vi "Autonomous Independent.vi"() -> ()   [LabVIEW 2020]
doc: "This VI is called when autonomous begins, and will automatically be terminated when autonomous ends. You can carry out timed or sensor driven robot movement independently without needing to return to the caller."
uses:
  <vilib>/Rock Robotics/WPI/ThirdParty/REV Robotics/REVLib/Typedef/Spark MAX Sensor Type.ctl
  <vilib>/Rock Robotics/WPI/Utilities/WPI_GetSetVariantRefNum.vi
  <vilib>/Rock Robotics/Network Tables/NT Read String.vi
  <vilib>/Rock Robotics/Network Tables/NT Write Numeric Array.vi
  <vilib>/Rock Robotics/Network Tables/NT Write Number.vi
  Robot Global Data.vi
  <vilib>/Rock Robotics/WPI/RobotDrive/WPI_RobotDriveArcadeDrive_Standard(NoSaturation).vi
  <vilib>/Rock Robotics/WPI/Solenoid/WPI_SolenoidValue.ctl
  <vilib>/Rock Robotics/WPI/Solenoid/WPI_SolenoidSetEnum.vi
panel:
  out "Real Yaw 2":dbl
  out "Right Drive Encoder 3":dbl format="%#.3f"
  out "Sensor Position 3":dbl
  out "Timestamp 3":u32
  out "Right Drive Encoder 2":dbl format="%#.3f"
  out "Sensor Position 2":dbl
  out "Timestamp 2":u32
  out "Sensor Position":dbl
  out "Timestamp":u32
  in  "error in 2":errorcluster
  out "Real Yaw":dbl
  out "Right Drive Encoder":dbl format="%#.3f"
  in  "error in":errorcluster
  # "Be sure to right-click and choose Data Operations>>Make Current Value default if you want to save the array values with the VI"
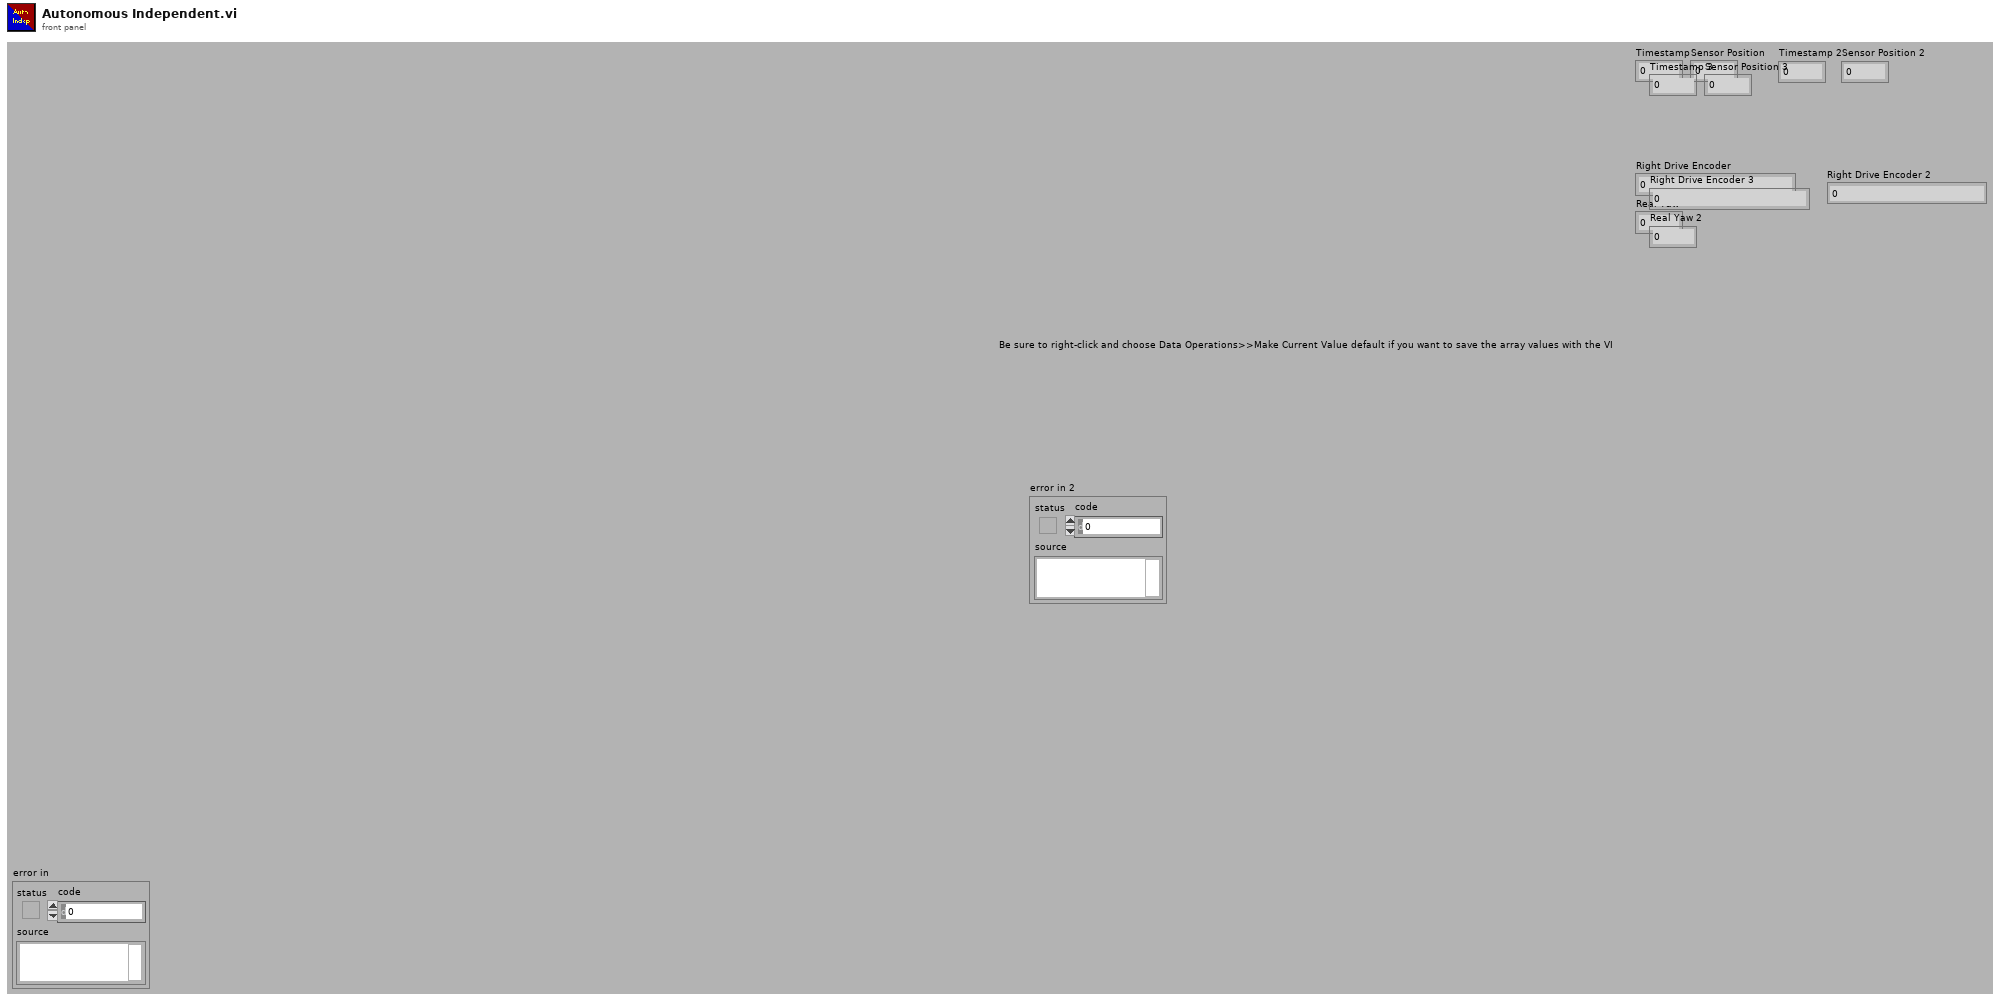
[diagram p1: front panel]
types:
  T1 = typedef "Spark MAX Sensor Type.ctl" = enum16{"No Sensor", "Hall Sensor", "Encoder", "-Not Available-", "Analog", "Alternate Encoder", "Duty Cycle"}
  T2 = typedef "WPI_JoystickDevRef.ctl" = cluster{"Device":T3}
  T3 = typedef "WPI_JoystickDeviceEnum.ctl" = enum16{"USB 0", "USB 1", "USB 2", "USB 3", "USB 4", "USB 5"}
  T4 = typedef "WPI_RobotDriveDevRef.ctl" = cluster{"DevStatus":errorcluster, "Motors[]":T5[], "Square Inputs":bool, "Max Output":dbl}
  T5 = typedef "WPI_MotorControlDeviceRef.ctl" = cluster{"DeviceStatus":errorcluster, "Type":T6, "PWM":cluster{"PWM Channel":T7, "DeadBand":T8}, "CAN":cluster{"Device Number":u8, "SetOutput VI Ref":variant, "GetOutput VI Ref":variant, "Enable VI Ref":variant, "Disable VI Ref":variant, "Data":variant}, "Invert":bool, "DIO PWM":cluster{"PWM \"Enable\" Channel":T7, "DIOChannel":T9, "PWM Rate":dbl}}
  T6 = typedef "WPI_MotorControlType.ctl" = enum16{"PWM", "CAN", "DIO PWM"}
  T7 = typedef "FPGA_DIOPWMChannel.ctl" = enum8{"PWM 0", "PWM 1", "PWM 2", "PWM 3", "PWM 4", "PWM 5", "PWM 6", "PWM 7", "PWM 8", "PWM 9", "PWM MXP 0", "PWM MXP 1", "PWM MXP 2", "PWM MXP 3", "PWM MXP 4", "PWM MXP 5", "PWM MXP 6", "PWM MXP 7", "PWM MXP 8", "PWM MXP 9", "Invalid"}
  T8 = typedef "WPI_PWMDeadband.ctl" = cluster{"Name":string, "maxPositivePwm":i32, "minPositivePwm":i32, "centerPwm":i32, "maxNegativePwm":i32, "minNegativePwm":i32, "angularRange":u16}
  T9 = typedef "FPGA_DIOChannel.ctl" = enum8{"DIO 0", "DIO 1", "DIO 2", "DIO 3", "DIO 4", "DIO 5", "DIO 6", "DIO 7", "DIO 8", "DIO 9", "DIO MXP 0", "DIO MXP 1", "DIO MXP 2", "DIO MXP 3", "DIO MXP 4", "DIO MXP 5", "DIO MXP 6", "DIO MXP 7", "DIO MXP 8", "DIO MXP 9", "DIO MXP 10", "DIO MXP 11", "DIO MXP 12", "DIO MXP 13", "DIO MXP 14", "DIO MXP 15", "SPI Port CS1", "SPI Port CS2", "SPI Port CS3", "SPI Port MISO", "SPI Port MOSI", "Invalid"}
  T10 = cluster{"Motors[][0]":T5, "Motors[][1]":T5, "Motors[][2]":T5, "Motors[][3]":T5, "Motors[][4]":T5, "Motors[][5]":T5, "Motors[][6]":T5, "Motors[][7]":T5, "Motors[][8]":T5}
  T11 = typedef "WPI_SolenoidValue.ctl" = enum16{"Off", "On", "Forward", "Reverse"}
  T12 = typedef "WPI_SolenoidDevRef.ctl" = cluster{"DevStatus":errorcluster, "Pneumatics Control Module":u8, "Forward Solenoid Channel":T13, "Reverse Solenoid Channel":T13}
  T13 = typedef "WPI_SolenoidChannel.ctl" = enum8{"Solenoid 0", "Solenoid 1", "Solenoid 2", "Solenoid 3", "Solenoid 4", "Solenoid 5", "Solenoid 6", "Solenoid 7", "Solenoid 8", "Solenoid 9", "Solenoid 10", "Solenoid 11", "Solenoid 12", "Solenoid 13", "Solenoid 14", "Solenoid 15", "Invalid"}
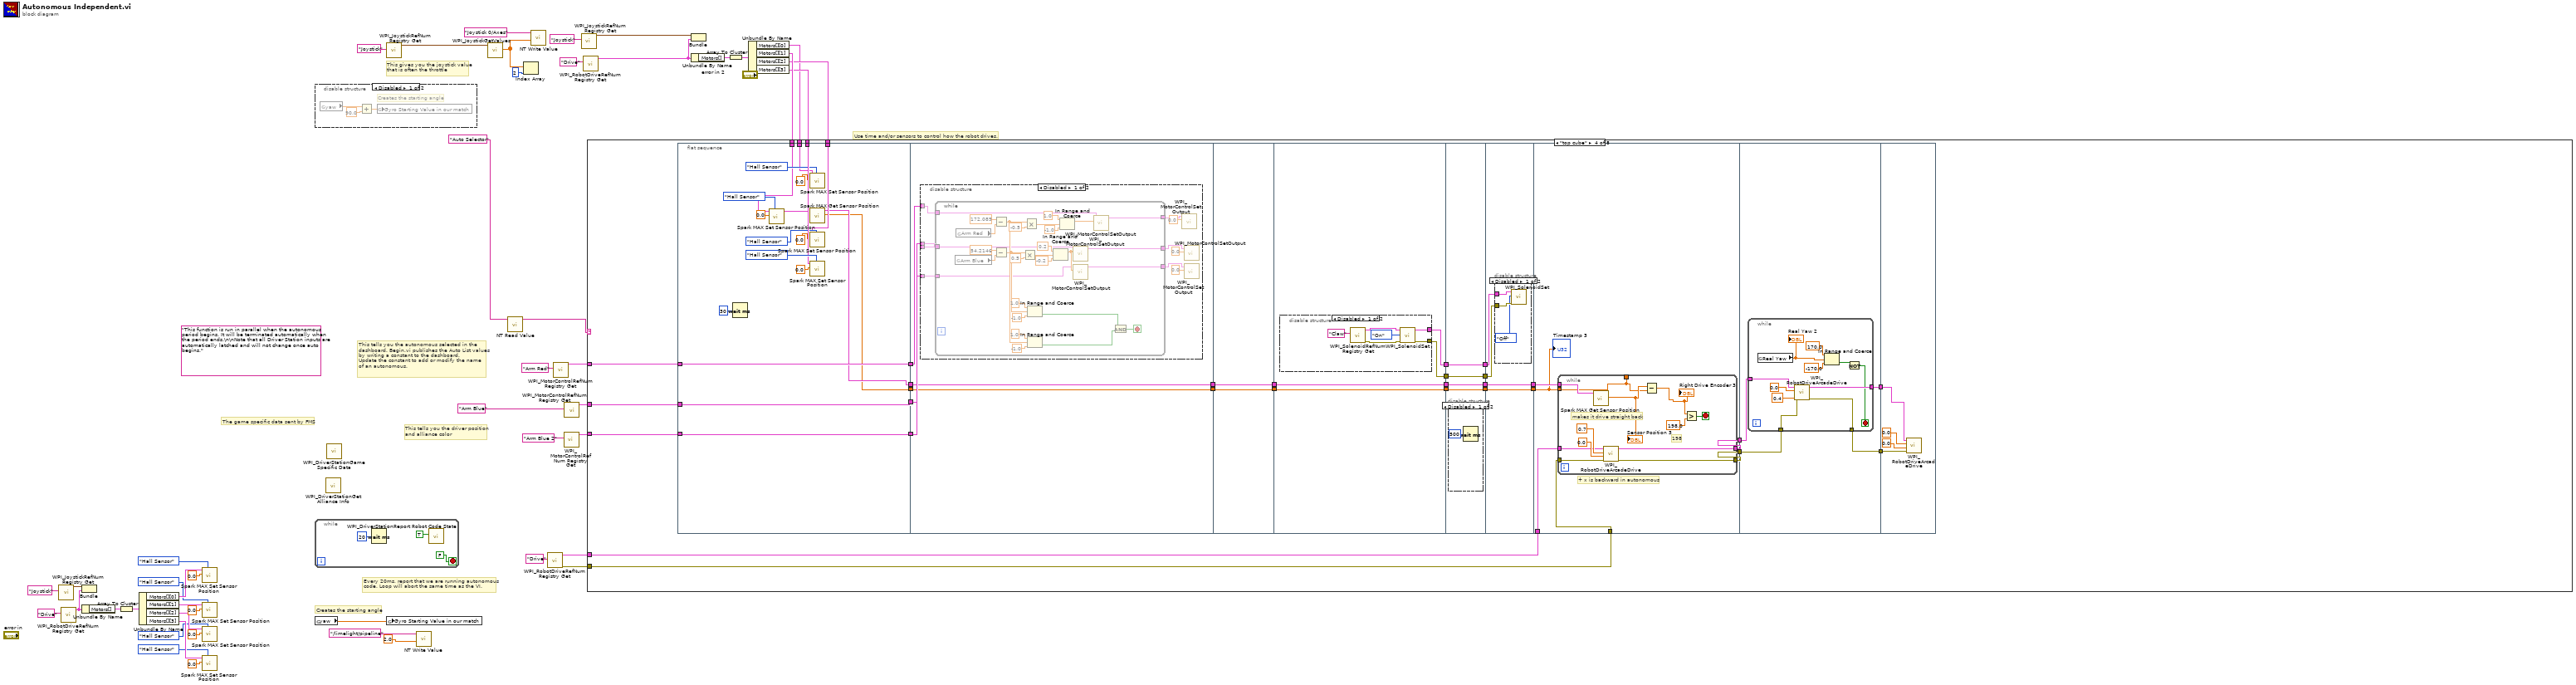
[diagram p0: block diagram]
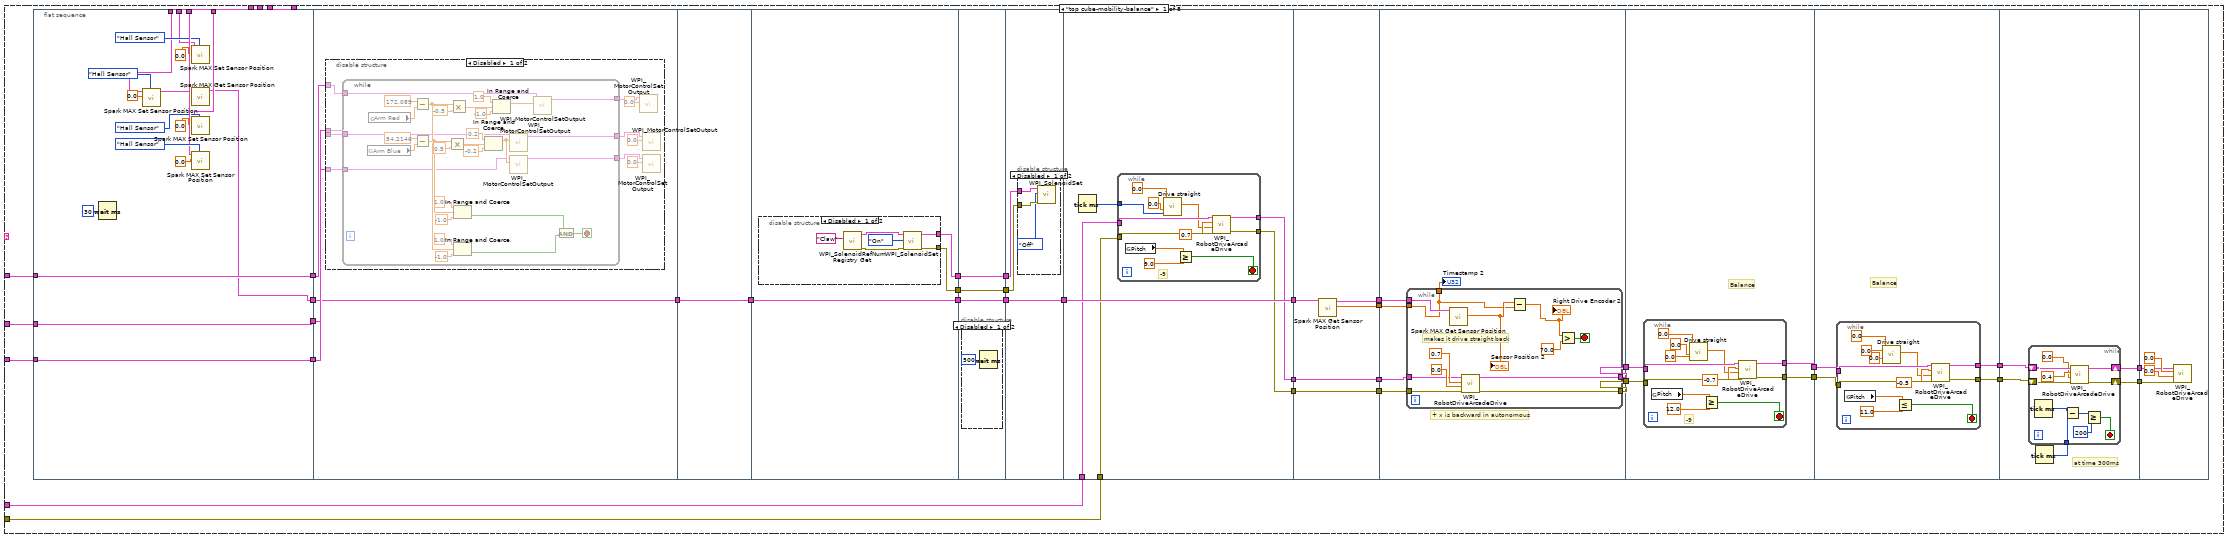
[diagram p3: hidden frame]
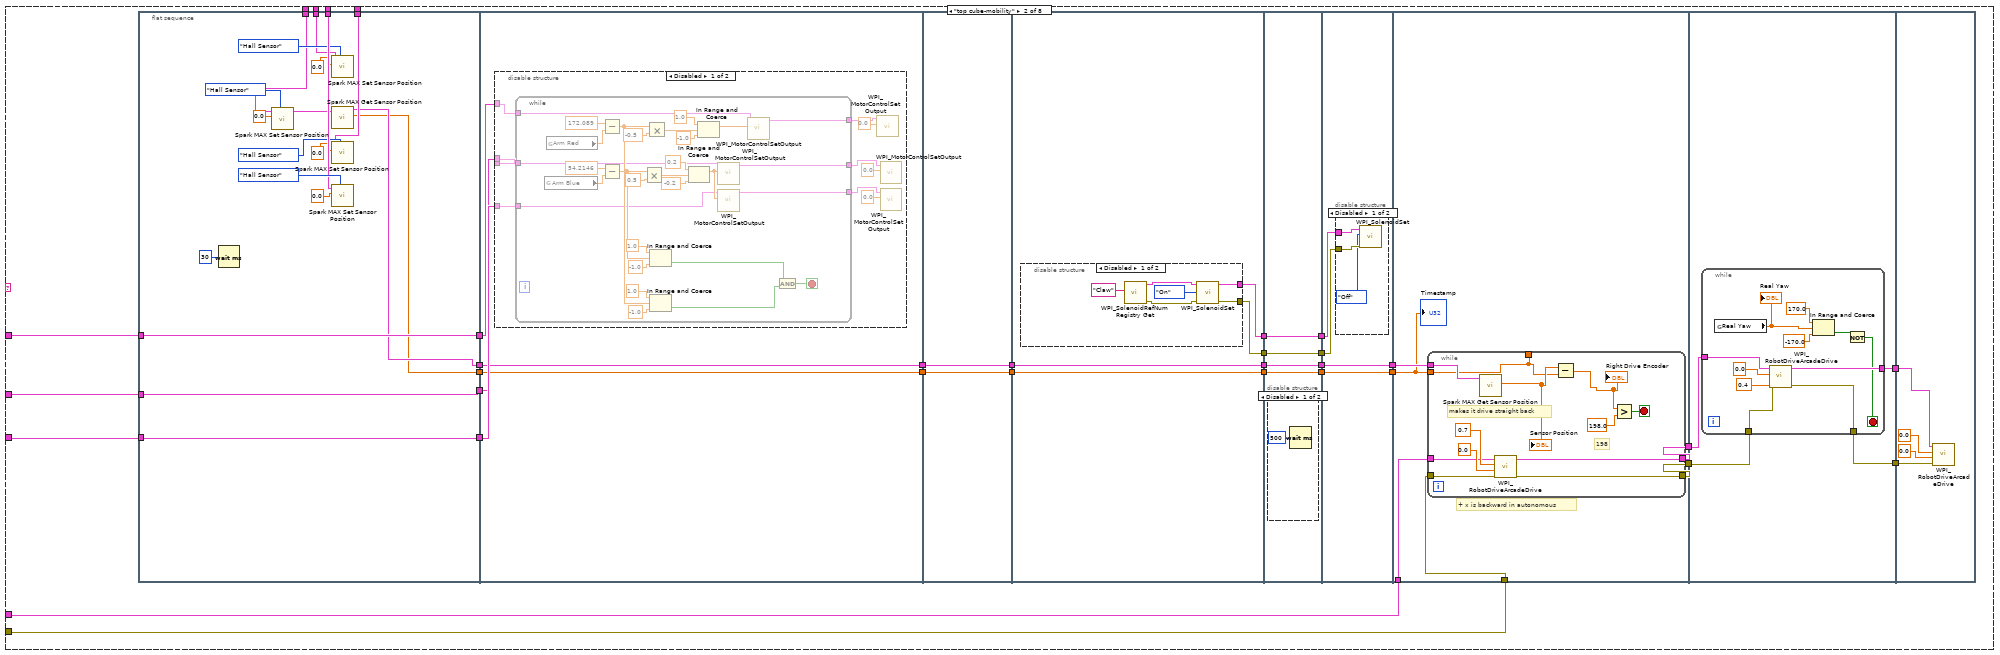
[diagram p8: hidden frame]
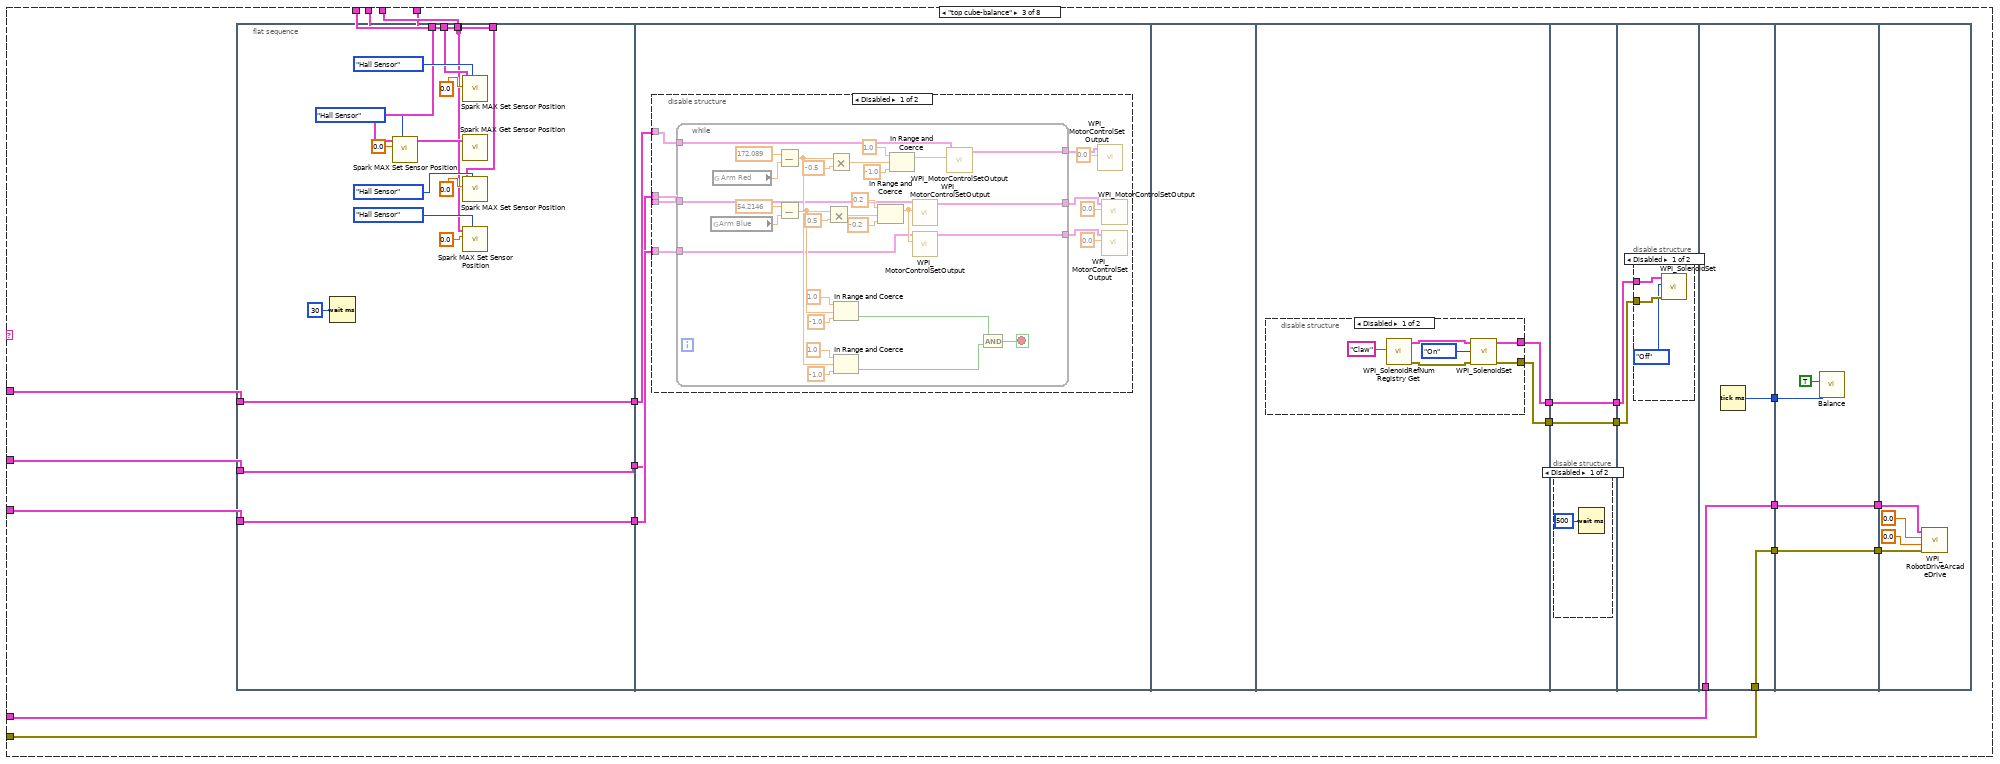
[diagram p13: hidden frame]
diagram:
  (unwired) "This function is run in parallel when the autonomous period begins. It will be terminated automatically when the period ends.\n\nNote that all Driver Station inputs are automatically latched and will not change once auto begins."
  # "Creates the starting angle"
  # "The game specific data sent by FMS"
  # "This tells you the autonomous selected in the \ndashboard. Begin.vi publishes the Auto List values\nby writing a constant to the dashboard.\nUpdate the constant to add or modify the name\nof an autonomous."
  # "Every 20ms, report that we are running autonomous\ncode. Loop will abort the same time as the VI."
  # "This gives you the joystick value\nthat is often the throttle"
  # "Use time and/or sensors to control how the robot drives."
  # "This tells you the driver position\nand alliance color"
  n1 = call <vilib>:"WPI_JoystickRefNum Registry Get.vi"("refnum name"="Joystick") -> ("JoystickDevRef"=w26:T2)  [unwired: 1 in, 9 out]
  n2 = call <vilib>:"WPI_RobotDriveRefNum Registry Get.vi"("refnum name"="Drive") -> ("RobotDriveDevRef"=w22:T4)  [unwired: 1 in, 9 out]
  n3 = Bundle("JoystickDevRef"=w26, "RobotDriveDevRef"=w22) -> ()  [unwired: 2 out]
  n4 = Unbundle By Name(w22) -> ("Motors[]"=w25:T5[])
  n5 = Array To Cluster(array=w25) -> (cluster=w24:T10)
  n6 = Unbundle By Name(w24) -> ("Motors[][0]"=w21:T5, "Motors[][1]"=w20:T5, "Motors[][2]"=w19:T5, "Motors[][3]"=w18:T5)
  n7 = call <vilib>:"Spark MAX Set Sensor Position.vi"("Sensor Type (Hall Sensor)"=Spark_MAX_Sensor_Type."Hall Sensor", "Position"=0.0, "MotorControlDeviceRef"=w21) -> ()  [unwired: 7 in, 2 out]
  n8 = call <vilib>:"Spark MAX Set Sensor Position.vi"("Sensor Type (Hall Sensor)"=Spark_MAX_Sensor_Type."Hall Sensor", "Position"=0.0, "MotorControlDeviceRef"=w20) -> ()  [unwired: 7 in, 2 out]
  n9 = call <vilib>:"Spark MAX Set Sensor Position.vi"("Sensor Type (Hall Sensor)"=Spark_MAX_Sensor_Type."Hall Sensor", "Position"=0.0, "MotorControlDeviceRef"=w19) -> ()  [unwired: 7 in, 2 out]
  n10 = call <vilib>:"Spark MAX Set Sensor Position.vi"("Sensor Type (Hall Sensor)"=Spark_MAX_Sensor_Type."Hall Sensor", "Position"=0.0, "MotorControlDeviceRef"=w18) -> ()  [unwired: 7 in, 2 out]
  n11 = disable-structure shown="Disabled" {
    frame Disabled {
      # "Creates the starting angle"
      n12 = global read "Robot Global Data.vi" "yaw"() -> (w49:dbl)
      n13 = Add(x=w49, y=90.0) -> (x+y=w50:dbl)
      n14 = global write "Robot Global Data.vi" "Gyro Starting Value in our match"(w50) -> ()
    }
    frame Enabled {
    }
  }
  n15 = while {
    stop <- FALSE stop-if-true
    n16 = Wait (ms)(milliseconds to wait=u32 20) -> ()  [unwired: 1 out]
    n17 = call <vilib>:"WPI_DriverStationReport Robot Code State.vi"("Autonomous"=TRUE) -> ()  [unwired: 10 in, 1 out]
  }
  n18 = global read "Robot Global Data.vi" "yaw"() -> (w40:dbl)
  n19 = call <vilib>:"WPI_DriverStationGet Alliance Info.vi"() -> ()  [unwired: 12 out]
  n20 = call <vilib>:"WPI_DriverStationGame Specific Data.vi"() -> ()  [unwired: 11 in, 1 out]
  n21 = call <vilib>:"WPI_JoystickRefNum Registry Get.vi"("refnum name"="Joystick") -> ("JoystickDevRef"=w46:T2)  [unwired: 1 in, 9 out]
  n22 = global write "Robot Global Data.vi" "Gyro Starting Value in our match"(w40) -> ()
  n23 = call-poly <vilib>:"NT Write Value.vi"("value"=2.0, "name"="/limelight/pipeline" ("Name")) -> ()  [unwired: 9 in, 1 out]
  n24 = call <vilib>:"WPI_JoystickGetValues.vi"("JoystickDevRef"=w46) -> ("Axes"=w42:dbl[])  [unwired: 6 in, 4 out]
  n25 = call-poly <vilib>:"NT Read Value.vi"("name"="Auto Selector" ("Name")) -> ("value"=w43:string)  [unwired: 8 in, 2 out]
  n26 = Index Array(array=w42, index=2) -> ()  [unwired: 1 out]
  n27 = call-poly <vilib>:"NT Write Value.vi"("value"=w42, "name"="Joystick 0/Axes" ("Name")) -> ()  [unwired: 9 in, 1 out]
  n28 = call <vilib>:"WPI_RobotDriveRefNum Registry Get.vi"("refnum name"="Drive") -> ("error out"=w29:errorcluster, "RobotDriveDevRef"=w30:T4)  [unwired: 9 in]
  n29 = call <vilib>:"WPI_MotorControlRefNum Registry Get.vi"("refnum name"="Arm Red") -> ("MotorControlDevRef"=w34:T5)  [unwired: 9 in, 1 out]
  n30 = call <vilib>:"WPI_MotorControlRefNum Registry Get.vi"("refnum name"="Arm Blue 2") -> ("MotorControlDevRef"=w32:T5)  [unwired: 9 in, 1 out]
  n31 = call <vilib>:"WPI_MotorControlRefNum Registry Get.vi"("refnum name"="Arm Blue") -> ("MotorControlDevRef"=w33:T5)  [unwired: 9 in, 1 out]
  n32 = call <vilib>:"WPI_JoystickRefNum Registry Get.vi"("refnum name"="Joystick") -> ("JoystickDevRef"=w7:T2)  [unwired: 1 in, 9 out]
  n33 = call <vilib>:"WPI_RobotDriveRefNum Registry Get.vi"("refnum name"="Drive") -> ("RobotDriveDevRef"=w10:T4)  [unwired: 1 in, 9 out]
  n34 = Bundle("JoystickDevRef"=w7, "RobotDriveDevRef"=w10) -> ()  [unwired: 2 out]
  n35 = Unbundle By Name(w10) -> ("Motors[]"=w8:T5[])
  n36 = Array To Cluster(array=w8) -> (cluster=w9:T10)
  n37 = Unbundle By Name(w9) -> ("Motors[][0]"=w1:T5, "Motors[][1]"=w4:T5, "Motors[][2]"=w2:T5, "Motors[][3]"=w3:T5)
  n38 = case shown="\"top cube\"" w43 {
    tunnel: w34 -> [w90 w296 w433 w557 _ _ _ _]
    tunnel: w33 -> [w89 w295 w432 w556 _ _ _ _]
    tunnel: w32 -> [w88 w294 w431 w555 _ _ _ _]
    tunnel: w30 -> [w70 w289 w430 w550 _ w686 w715 _]
    tunnel: w29 -> [w69 w288 w429 w549 _ w685 w714 _]
    tunnel: w4 -> [w75 w274 w427 w535 _ _ _ _]
    tunnel: w3 -> [w74 w273 w425 w534 _ _ _ _]
    tunnel: w2 -> [w73 w272 w424 w533 _ _ _ _]
    tunnel: w1 -> [w72 w271 w426 w532 _ _ _ _]
    frame "top cube-mobility-balance" {
      n39 = flat-sequence {
        tunnel: w88 -> [w108]
        tunnel: w89 -> [w107]
        tunnel: w90 -> [w106]
        tunnel: [w108] -> w83
        tunnel: [w96] -> w78
        tunnel: [w107] -> w77
        tunnel: [w106] -> w76
        tunnel: w75 -> [w94]
        tunnel: w74 -> [w103]
        tunnel: w73 -> [w100]
        tunnel: w72 -> [w97]
        tunnel: w83 -> [w112]
        tunnel: [w111] -> w79
        tunnel: w78 -> [w111]
        tunnel: w77 -> [w109]
        tunnel: w76 -> [w110]
        tunnel: [w151] -> w80
        tunnel: w79 -> [w151]
        tunnel: [w154] -> w87
        tunnel: [w153] -> w85
        tunnel: [w152] -> w81
        tunnel: w80 -> [w152]
        tunnel: w87 -> [w163]
        tunnel: [w163] -> w86
        tunnel: w85 -> [w162]
        tunnel: [w162] -> w84
        tunnel: [w161] -> w82
        tunnel: w81 -> [w161]
        tunnel: w86 -> [w167]
        tunnel: w84 -> [w166]
        tunnel: [w165] -> w71
        tunnel: w82 -> [w165]
        tunnel: w71 -> [w176]
        tunnel: [w176] -> w66
        tunnel: w70 -> [w174]
        tunnel: w69 -> [w173]
        tunnel: [w172] -> w64
        tunnel: [w171] -> w62
        tunnel: w66 -> [w191]
        tunnel: [w190] -> w65
        tunnel: w64 -> [w193]
        tunnel: [w193] -> w63
        tunnel: w62 -> [w192]
        tunnel: [w192] -> w61
        tunnel: [w189] -> w60
        tunnel: [w200] -> w68
        tunnel: [w199] -> w67
        tunnel: w65 -> [w198]
        tunnel: w63 -> [w197]
        tunnel: w61 -> [w196]
        tunnel: w60 -> [w195]
        tunnel: w68 -> [w216]
        tunnel: [w214] -> w59
        tunnel: w67 -> [w215]
        tunnel: [w213] -> w58
        tunnel: w59 -> [w232]
        tunnel: w58 -> [w231]
        tunnel: [w230] -> w57
        tunnel: [w229] -> w56
        tunnel: w57 -> [w248]
        tunnel: w56 -> [w247]
        tunnel: [w246] -> w55
        tunnel: [w245] -> w54
        tunnel: w55 -> [w262]
        tunnel: w54 -> [w261]
        frame #0 {
          n40 = Wait (ms)(milliseconds to wait=u32 30) -> ()  [unwired: 1 out]
          n41 = call <vilib>:"Spark MAX Set Sensor Position.vi"("Sensor Type (Hall Sensor)"=Spark_MAX_Sensor_Type."Hall Sensor", "Position"=0.0, "MotorControlDeviceRef"=w94) -> ("MotorControlDeviceRef"=w93:T5)  [unwired: 7 in, 1 out]
          n42 = call <vilib>:"Spark MAX Set Sensor Position.vi"("Sensor Type (Hall Sensor)"=Spark_MAX_Sensor_Type."Hall Sensor", "Position"=0.0, "MotorControlDeviceRef"=w97) -> ()  [unwired: 7 in, 2 out]
          n43 = call <vilib>:"Spark MAX Get Sensor Position.vi"("MotorControlDevRef in"=w93) -> ("MotorControlDevRef out"=w96:T5)  [unwired: 7 in, 3 out]
          n44 = call <vilib>:"Spark MAX Set Sensor Position.vi"("Sensor Type (Hall Sensor)"=Spark_MAX_Sensor_Type."Hall Sensor", "Position"=0.0, "MotorControlDeviceRef"=w100) -> ()  [unwired: 7 in, 2 out]
          n45 = call <vilib>:"Spark MAX Set Sensor Position.vi"("Sensor Type (Hall Sensor)"=Spark_MAX_Sensor_Type."Hall Sensor", "Position"=0.0, "MotorControlDeviceRef"=w103) -> ()  [unwired: 7 in, 2 out]
        }
        frame #1 {
          n46 = disable-structure shown="Disabled" {
            disable-tunnel: w110 -> [w121 _]
            disable-tunnel: [w113 _] -> _
            disable-tunnel: w112 -> [w120 _]
            disable-tunnel: w109 -> [w113 _]
            frame Disabled {
              n47 = while {
                tunnel: w121 -> [w127]
                tunnel: w113 -> [w126]
                tunnel: w120 -> [w125]
                tunnel: [w122] -> w119
                tunnel: [w124] -> w118
                tunnel: [w123] -> w117
                stop <- w150 stop-if-true
                n48 = global read "Robot Global Data.vi" "Arm Blue"() -> (w130:dbl)
                n49 = global read "Robot Global Data.vi" "Arm Red"() -> (w141:dbl)
                n50 = Subtract(x=172.089, y=w141) -> (x-y=w128:dbl)
                n51 = Subtract(x=54.2146, y=w130) -> (x-y=w129:dbl)
                n52 = Multiply(x=w129, y=0.5) -> (x*y=w138:dbl)
                n53 = Multiply(x=w128, y=-0.5) -> (x*y=w137:dbl)
                n54 = In Range and Coerce(upper limit=1.0, x=w129, lower limit=-1.0) -> (In Range?=w149:bool)  [unwired: 1 out]
                n55 = In Range and Coerce(upper limit=1.0, x=w128, lower limit=-1.0) -> (In Range?=w148:bool)  [unwired: 1 out]
                n56 = In Range and Coerce(upper limit=0.2, x=w138, lower limit=-0.2) -> (coerced(x)=w133:dbl)  [unwired: 1 out]
                n57 = In Range and Coerce(upper limit=1.0, x=w137, lower limit=-1.0) -> (coerced(x)=w134:dbl)  [unwired: 1 out]
                n58 = call <vilib>:"WPI_MotorControlSetOutput.vi"("Output"=w133, "MotorControlDevRef"=w126) -> ("MotorControlDevRef"=w122:T5)  [unwired: 7 in, 2 out]
                n59 = call <vilib>:"WPI_MotorControlSetOutput.vi"("Output"=w133, "MotorControlDevRef"=w125) -> ("MotorControlDevRef"=w124:T5)  [unwired: 7 in, 2 out]
                n60 = call <vilib>:"WPI_MotorControlSetOutput.vi"("Output"=w134, "MotorControlDevRef"=w127) -> ("MotorControlDevRef"=w123:T5)  [unwired: 7 in, 2 out]
                n61 = And(x=w149, y=w148) -> (x .and. y?=w150:bool)
              }
              n62 = call <vilib>:"WPI_MotorControlSetOutput.vi"("Output"=0.0, "MotorControlDevRef"=w117) -> ()  [unwired: 7 in, 3 out]
              n63 = call <vilib>:"WPI_MotorControlSetOutput.vi"("Output"=0.0, "MotorControlDevRef"=w119) -> ()  [unwired: 7 in, 3 out]
              n64 = call <vilib>:"WPI_MotorControlSetOutput.vi"("Output"=0.0, "MotorControlDevRef"=w118) -> ()  [unwired: 7 in, 3 out]
            }
            frame Enabled {
            }
          }
        }
        frame #2 {
        }
        frame #3 {
          n65 = disable-structure shown="Disabled" {
            disable-tunnel: [w156 _] -> w154
            disable-tunnel: [w155 _] -> w153
            frame Disabled {
              n66 = call <vilib>:"WPI_SolenoidRefNum Registry Get.vi"("refnum name"="Claw") -> ("error out"=w160:errorcluster, "SolenoidDevRef"=w159:T12)  [unwired: 9 in]
              n67 = call-poly <vilib>:"WPI_SolenoidSet.vi"("error in (no error)"=w160, "Value"=WPI_SolenoidValue."On", "SolenoidDevRef"=w159) -> ("error out"=w155:errorcluster, "SolenoidDevRef"=w156:T12)  [unwired: 7 in]
            }
            frame Enabled {
            }
          }
        }
        frame #4 {
          n68 = disable-structure shown="Disabled" {
            frame Disabled {
              n69 = Wait (ms)(milliseconds to wait=u32 500) -> ()  [unwired: 1 out]
            }
            frame Enabled {
            }
          }
        }
        frame #5 {
          n70 = disable-structure shown="Disabled" {
            disable-tunnel: w167 -> [w170 _]
            disable-tunnel: w166 -> [w169 _]
            frame Disabled {
              n71 = call-poly <vilib>:"WPI_SolenoidSet.vi"("error in (no error)"=w169, "Value"=WPI_SolenoidValue."Off", "SolenoidDevRef"=w170) -> ()  [unwired: 7 in, 2 out]
            }
            frame Enabled {
            }
          }
        }
        frame #6 {
          n72 = Tick Count (ms)() -> (millisecond timer value=w175:u32)
          n73 = while {
            tunnel: [w186] -> w172
            tunnel: w174 -> [w185]
            tunnel: w173 -> [w184]
            tunnel: [w182] -> w171
            tunnel: w175 -> [w178]
            stop <- w188 stop-if-true
            # "-9"
            n74 = global read "Robot Global Data.vi" "Pitch"() -> (w183:dbl)
            n75 = call "Drive straight.vi"("Start Time"=w178, "Length(seconds)"=0.0, "Desired angle"=0.0) -> ("X Power"=w179:dbl)  [unwired: 7 in, 1 out]
            n76 = Greater Or Equal?(x=w183, y=9.0) -> (x >= y?=w188:bool)
            n77 = call-poly <vilib>:"WPI_RobotDriveArcadeDrive.vi"("error in (no error)"=w184, "Y axis value"=w179, "X axis value"=0.7 ("Y axis value"), "RobotDriveDevRef"=w185) -> ("error out"=w182:errorcluster, "RobotDriveDevRef"=w186:T4)  [unwired: 5 in, 1 out]
          }
        }
        frame #7 {
          n78 = call <vilib>:"Spark MAX Get Sensor Position.vi"("MotorControlDevRef in"=w191) -> ("Sensor Position"=w189:dbl, "MotorControlDevRef out"=w190:T5)  [unwired: 7 in, 2 out]
        }
        frame #8 {
          # "+ x is backward in autonomous"
          n79 = while {
            tunnel: [w210] -> w200
            tunnel: [w209] -> w199
            tunnel: w197 -> [w207]
            tunnel: w198 -> [w205]
            tunnel: w196 -> [w202]
            tunnel: w195 -> [w201]
            tunnel: [w201] -> w194
            stop <- w208 stop-if-true
            # "makes it drive straight back"
            n80 = call <vilib>:"Spark MAX Get Sensor Position.vi"("MotorControlDevRef in"=w205) -> ("Sensor Position"=w203:dbl)  [unwired: 7 in, 3 out]
            "Sensor Position 2" <- w203
            n81 = call-poly <vilib>:"WPI_RobotDriveArcadeDrive.vi"("error in (no error)"=w202, "Y axis value"=0.0, "X axis value"=0.7, "RobotDriveDevRef"=w207) -> ("error out"=w209:errorcluster, "RobotDriveDevRef"=w210:T4)  [unwired: 5 in, 1 out]
            n82 = Subtract(x=w203, y=w201) -> (x-y=w204:dbl)
            "Right Drive Encoder 2" <- w204
            n83 = Greater?(x=w204, y=70.0) -> (0:w208:bool)
          }
          "Timestamp 2" <- w194
        }
        frame #9 {
          # "Balance"
          n84 = while {
            tunnel: [w226] -> w214
            tunnel: w216 -> [w225]
            tunnel: w215 -> [w224]
            tunnel: [w222] -> w213
            stop <- w228 stop-if-true
            # "-9"
            n85 = global read "Robot Global Data.vi" "Pitch"() -> (w223:dbl)
            n86 = call "Drive straight.vi"("Start Time"=0.0, "Length(seconds)"=0.0, "Desired angle"=0.0) -> ("X Power"=w219:dbl)  [unwired: 7 in, 1 out]
            n87 = Greater Or Equal?(x=w223, y=12.0) -> (x >= y?=w228:bool)
            n88 = call-poly <vilib>:"WPI_RobotDriveArcadeDrive.vi"("error in (no error)"=w224, "Y axis value"=w219, "X axis value"=-0.7 ("Y axis value"), "RobotDriveDevRef"=w225) -> ("error out"=w222:errorcluster, "RobotDriveDevRef"=w226:T4)  [unwired: 5 in, 1 out]
          }
        }
        frame #10 {
          # "Balance"
          n89 = while {
            tunnel: [w242] -> w230
            tunnel: w232 -> [w241]
            tunnel: w231 -> [w240]
            tunnel: [w238] -> w229
            stop <- w244 stop-if-true
            n90 = global read "Robot Global Data.vi" "Pitch"() -> (w239:dbl)
            n91 = call "Drive straight.vi"("Start Time"=0.0, "Length(seconds)"=0.0, "Desired angle"=0.0) -> ("X Power"=w234:dbl)  [unwired: 7 in, 1 out]
            n92 = Less Or Equal?(x=w239, y=11.0) -> (x <= y?=w244:bool)
            n93 = call-poly <vilib>:"WPI_RobotDriveArcadeDrive.vi"("error in (no error)"=w240, "Y axis value"=w234, "X axis value"=-0.5 ("Y axis value"), "RobotDriveDevRef"=w241) -> ("error out"=w238:errorcluster, "RobotDriveDevRef"=w242:T4)  [unwired: 5 in, 1 out]
          }
        }
        frame #11 {
          # "at time 300ms"
          n94 = Tick Count (ms)() -> (millisecond timer value=w249:u32)
          n95 = while {
            shift-right: [w258] -> w246
            shift-left: w248 -> [w260]
            shift-right: [w257] -> w245
            shift-left: w247 -> [w259]
            tunnel: w249 -> [w255]
            stop <- w252 stop-if-true
            n96 = Tick Count (ms)() -> (millisecond timer value=w256:u32)
            n97 = Subtract(x=w256, y=w255) -> (x-y=w254:u32)
            n98 = call-poly <vilib>:"WPI_RobotDriveArcadeDrive.vi"("error in (no error)"=w259, "Y axis value"=0.0 ("X axis value"), "X axis value"=0.4 ("Y axis value"), "RobotDriveDevRef"=w260) -> ("error out"=w257:errorcluster, "RobotDriveDevRef"=w258:T4)  [unwired: 5 in, 1 out]
            n99 = Greater Or Equal?(x=w254, y=u32 200) -> (x >= y?=w252:bool)
          }
        }
        frame #12 {
          n100 = call-poly <vilib>:"WPI_RobotDriveArcadeDrive.vi"("error in (no error)"=w261, "Y axis value"=0.0, "X axis value"=0.0, "RobotDriveDevRef"=w262) -> ()  [unwired: 5 in, 3 out]
        }
      }
    }
    frame "top cube-mobility" {
      n101 = flat-sequence {
        tunnel: w294 -> [w315]
        tunnel: w295 -> [w314]
        tunnel: w296 -> [w313]
        tunnel: [w315] -> w283
        tunnel: [w303] -> w277
        tunnel: [w314] -> w276
        tunnel: [w313] -> w275
        tunnel: w274 -> [w300]
        tunnel: w273 -> [w310]
        tunnel: w272 -> [w307]
        tunnel: w271 -> [w304]
        tunnel: [w302] -> w265
        tunnel: w283 -> [w320]
        tunnel: [w319] -> w278
        tunnel: w277 -> [w319]
        tunnel: w276 -> [w317]
        tunnel: w275 -> [w318]
        tunnel: [w316] -> w266
        tunnel: w265 -> [w316]
        tunnel: [w360] -> w279
        tunnel: w278 -> [w360]
        tunnel: [w359] -> w267
        tunnel: w266 -> [w359]
        tunnel: [w364] -> w293
        tunnel: [w363] -> w291
        tunnel: [w362] -> w280
        tunnel: w279 -> [w362]
        tunnel: [w361] -> w268
        tunnel: w267 -> [w361]
        tunnel: w293 -> [w374]
        tunnel: [w374] -> w292
        tunnel: w291 -> [w373]
        tunnel: [w373] -> w290
        tunnel: [w372] -> w281
        tunnel: w280 -> [w372]
        tunnel: [w371] -> w269
        tunnel: w268 -> [w371]
        tunnel: w292 -> [w379]
        tunnel: w290 -> [w378]
        tunnel: [w377] -> w282
        tunnel: w281 -> [w377]
        tunnel: [w376] -> w270
        tunnel: w269 -> [w376]
        tunnel: [w388] -> w287
        tunnel: [w387] -> w286
        tunnel: w289 -> [w386]
        tunnel: w288 -> [w385]
        tunnel: w282 -> [w384]
        tunnel: w270 -> [w383]
        tunnel: w287 -> [w404]
        tunnel: w286 -> [w403]
        tunnel: [w402] -> w285
        tunnel: [w401] -> w284
        tunnel: w285 -> [w417]
        tunnel: w284 -> [w416]
        frame #0 {
          n102 = Wait (ms)(milliseconds to wait=u32 30) -> ()  [unwired: 1 out]
          n103 = call <vilib>:"Spark MAX Set Sensor Position.vi"("Sensor Type (Hall Sensor)"=Spark_MAX_Sensor_Type."Hall Sensor", "Position"=0.0, "MotorControlDeviceRef"=w300) -> ("MotorControlDeviceRef"=w299:T5)  [unwired: 7 in, 1 out]
          n104 = call <vilib>:"Spark MAX Set Sensor Position.vi"("Sensor Type (Hall Sensor)"=Spark_MAX_Sensor_Type."Hall Sensor", "Position"=0.0, "MotorControlDeviceRef"=w304) -> ()  [unwired: 7 in, 2 out]
          n105 = call <vilib>:"Spark MAX Get Sensor Position.vi"("MotorControlDevRef in"=w299) -> ("Sensor Position"=w302:dbl, "MotorControlDevRef out"=w303:T5)  [unwired: 7 in, 2 out]
          n106 = call <vilib>:"Spark MAX Set Sensor Position.vi"("Sensor Type (Hall Sensor)"=Spark_MAX_Sensor_Type."Hall Sensor", "Position"=0.0, "MotorControlDeviceRef"=w307) -> ()  [unwired: 7 in, 2 out]
          n107 = call <vilib>:"Spark MAX Set Sensor Position.vi"("Sensor Type (Hall Sensor)"=Spark_MAX_Sensor_Type."Hall Sensor", "Position"=0.0, "MotorControlDeviceRef"=w310) -> ()  [unwired: 7 in, 2 out]
        }
        frame #1 {
          n108 = disable-structure shown="Disabled" {
            disable-tunnel: w318 -> [w329 _]
            disable-tunnel: [w321 _] -> _
            disable-tunnel: w320 -> [w328 _]
            disable-tunnel: w317 -> [w321 _]
            frame Disabled {
              n109 = while {
                tunnel: w329 -> [w335]
                tunnel: w321 -> [w334]
                tunnel: w328 -> [w333]
                tunnel: [w330] -> w327
                tunnel: [w332] -> w326
                tunnel: [w331] -> w325
                stop <- w358 stop-if-true
                n110 = global read "Robot Global Data.vi" "Arm Blue"() -> (w338:dbl)
                n111 = global read "Robot Global Data.vi" "Arm Red"() -> (w349:dbl)
                n112 = Subtract(x=172.089, y=w349) -> (x-y=w336:dbl)
                n113 = Subtract(x=54.2146, y=w338) -> (x-y=w337:dbl)
                n114 = Multiply(x=w337, y=0.5) -> (x*y=w346:dbl)
                n115 = Multiply(x=w336, y=-0.5) -> (x*y=w345:dbl)
                n116 = In Range and Coerce(upper limit=1.0, x=w337, lower limit=-1.0) -> (In Range?=w357:bool)  [unwired: 1 out]
                n117 = In Range and Coerce(upper limit=1.0, x=w336, lower limit=-1.0) -> (In Range?=w356:bool)  [unwired: 1 out]
                n118 = In Range and Coerce(upper limit=0.2, x=w346, lower limit=-0.2) -> (coerced(x)=w341:dbl)  [unwired: 1 out]
                n119 = In Range and Coerce(upper limit=1.0, x=w345, lower limit=-1.0) -> (coerced(x)=w342:dbl)  [unwired: 1 out]
                n120 = call <vilib>:"WPI_MotorControlSetOutput.vi"("Output"=w341, "MotorControlDevRef"=w334) -> ("MotorControlDevRef"=w330:T5)  [unwired: 7 in, 2 out]
                n121 = call <vilib>:"WPI_MotorControlSetOutput.vi"("Output"=w341, "MotorControlDevRef"=w333) -> ("MotorControlDevRef"=w332:T5)  [unwired: 7 in, 2 out]
                n122 = call <vilib>:"WPI_MotorControlSetOutput.vi"("Output"=w342, "MotorControlDevRef"=w335) -> ("MotorControlDevRef"=w331:T5)  [unwired: 7 in, 2 out]
                n123 = And(x=w357, y=w356) -> (x .and. y?=w358:bool)
              }
              n124 = call <vilib>:"WPI_MotorControlSetOutput.vi"("Output"=0.0, "MotorControlDevRef"=w325) -> ()  [unwired: 7 in, 3 out]
              n125 = call <vilib>:"WPI_MotorControlSetOutput.vi"("Output"=0.0, "MotorControlDevRef"=w327) -> ()  [unwired: 7 in, 3 out]
              n126 = call <vilib>:"WPI_MotorControlSetOutput.vi"("Output"=0.0, "MotorControlDevRef"=w326) -> ()  [unwired: 7 in, 3 out]
            }
            frame Enabled {
            }
          }
        }
        frame #2 {
        }
        frame #3 {
          n127 = disable-structure shown="Disabled" {
            disable-tunnel: [w366 _] -> w364
            disable-tunnel: [w365 _] -> w363
            frame Disabled {
              n128 = call <vilib>:"WPI_SolenoidRefNum Registry Get.vi"("refnum name"="Claw") -> ("error out"=w370:errorcluster, "SolenoidDevRef"=w369:T12)  [unwired: 9 in]
              n129 = call-poly <vilib>:"WPI_SolenoidSet.vi"("error in (no error)"=w370, "Value"=WPI_SolenoidValue."On", "SolenoidDevRef"=w369) -> ("error out"=w365:errorcluster, "SolenoidDevRef"=w366:T12)  [unwired: 7 in]
            }
            frame Enabled {
            }
          }
        }
        frame #4 {
          n130 = disable-structure shown="Disabled" {
            frame Disabled {
              n131 = Wait (ms)(milliseconds to wait=u32 500) -> ()  [unwired: 1 out]
            }
            frame Enabled {
            }
          }
        }
        frame #5 {
          n132 = disable-structure shown="Disabled" {
            disable-tunnel: w379 -> [w382 _]
            disable-tunnel: w378 -> [w381 _]
            frame Disabled {
              n133 = call-poly <vilib>:"WPI_SolenoidSet.vi"("error in (no error)"=w381, "Value"=WPI_SolenoidValue."Off", "SolenoidDevRef"=w382) -> ()  [unwired: 7 in, 2 out]
            }
            frame Enabled {
            }
          }
        }
        frame #6 {
          # "+ x is backward in autonomous"
          n134 = while {
            tunnel: [w398] -> w388
            tunnel: [w397] -> w387
            tunnel: w386 -> [w395]
            tunnel: w385 -> [w394]
            tunnel: w384 -> [w392]
            tunnel: w383 -> [w389]
            tunnel: [w389] -> _
            stop <- w396 stop-if-true
            # "198"
            # "makes it drive straight back"
            n135 = call <vilib>:"Spark MAX Get Sensor Position.vi"("MotorControlDevRef in"=w392) -> ("Sensor Position"=w390:dbl)  [unwired: 7 in, 3 out]
            "Sensor Position" <- w390
            n136 = call-poly <vilib>:"WPI_RobotDriveArcadeDrive.vi"("error in (no error)"=w394, "Y axis value"=0.0, "X axis value"=0.7, "RobotDriveDevRef"=w395) -> ("error out"=w397:errorcluster, "RobotDriveDevRef"=w398:T4)  [unwired: 5 in, 1 out]
            n137 = Subtract(x=w390, y=w389) -> (x-y=w391:dbl)
            "Right Drive Encoder" <- w391
            n138 = Greater?(x=w391, y=198.0) -> (0:w396:bool)
          }
          "Timestamp" <- w383
        }
        frame #7 {
          n139 = while {
            tunnel: w404 -> [w413]
            tunnel: w403 -> [w412]
            tunnel: [w411] -> w402
            tunnel: [w410] -> w401
            stop <- w405 stop-if-true
            n140 = global read "Robot Global Data.vi" "Real Yaw"() -> (w407:dbl)
            "Real Yaw" <- w407
            n141 = call-poly <vilib>:"WPI_RobotDriveArcadeDrive.vi"("error in (no error)"=w412, "Y axis value"=0.4, "X axis value"=0.0, "RobotDriveDevRef"=w413) -> ("error out"=w410:errorcluster, "RobotDriveDevRef"=w411:T4)  [unwired: 5 in, 1 out]
            n142 = In Range and Coerce(upper limit=170.0, x=w407, lower limit=-170.0) -> (In Range?=w406:bool)  [unwired: 1 out]
            n143 = Not(x=w406) -> (.not. x?=w405:bool)
          }
        }
        frame #8 {
          n144 = call-poly <vilib>:"WPI_RobotDriveArcadeDrive.vi"("error in (no error)"=w416, "Y axis value"=0.0, "X axis value"=0.0, "RobotDriveDevRef"=w417) -> ()  [unwired: 5 in, 3 out]
        }
      }
    }
    frame "top cube-balance" {
      n145 = flat-sequence {
        tunnel: w431 -> [w457]
        tunnel: w432 -> [w456]
        tunnel: w433 -> [w455]
        tunnel: [w457] -> w440
        tunnel: [w456] -> w439
        tunnel: [w455] -> w438
        tunnel: w427 -> [w445]
        tunnel: [w441] -> _
        tunnel: w424 -> [w450]
        tunnel: w426 -> [w447]
        tunnel: w425 -> [w441]
        tunnel: w440 -> [w460]
        tunnel: w439 -> [w458]
        tunnel: w438 -> [w459]
        tunnel: [w500] -> w437
        tunnel: [w499] -> w436
        tunnel: w437 -> [w508]
        tunnel: [w508] -> w435
        tunnel: w436 -> [w507]
        tunnel: [w507] -> w434
        tunnel: w435 -> [w511]
        tunnel: w434 -> [w510]
        tunnel: w430 -> [w516]
        tunnel: w429 -> [w515]
        tunnel: [w517] -> w428
        tunnel: [w516] -> w422
        tunnel: [w515] -> w420
        tunnel: w428 -> [w520]
        tunnel: [w519] -> w423
        tunnel: w422 -> [w519]
        tunnel: [w518] -> w421
        tunnel: w420 -> [w518]
        tunnel: w423 -> [w523]
        tunnel: w421 -> [w522]
        frame #0 {
          n146 = Wait (ms)(milliseconds to wait=u32 30) -> ()  [unwired: 1 out]
          n147 = call <vilib>:"Spark MAX Set Sensor Position.vi"("Sensor Type (Hall Sensor)"=Spark_MAX_Sensor_Type."Hall Sensor", "Position"=0.0, "MotorControlDeviceRef"=w445) -> ("MotorControlDeviceRef"=w444:T5)  [unwired: 7 in, 1 out]
          n148 = call <vilib>:"Spark MAX Set Sensor Position.vi"("Sensor Type (Hall Sensor)"=Spark_MAX_Sensor_Type."Hall Sensor", "Position"=0.0, "MotorControlDeviceRef"=w447) -> ()  [unwired: 7 in, 2 out]
          n149 = call <vilib>:"Spark MAX Get Sensor Position.vi"("MotorControlDevRef in"=w444) -> ()  [unwired: 7 in, 4 out]
          n150 = call <vilib>:"Spark MAX Set Sensor Position.vi"("Sensor Type (Hall Sensor)"=Spark_MAX_Sensor_Type."Hall Sensor", "Position"=0.0, "MotorControlDeviceRef"=w450) -> ()  [unwired: 7 in, 2 out]
          n151 = call <vilib>:"Spark MAX Set Sensor Position.vi"("Sensor Type (Hall Sensor)"=Spark_MAX_Sensor_Type."Hall Sensor", "Position"=0.0, "MotorControlDeviceRef"=w441) -> ()  [unwired: 7 in, 2 out]
        }
        frame #1 {
          n152 = disable-structure shown="Disabled" {
            disable-tunnel: w459 -> [w469 _]
            disable-tunnel: [w461 _] -> _
            disable-tunnel: w460 -> [w468 _]
            disable-tunnel: w458 -> [w461 _]
            frame Disabled {
              n153 = while {
                tunnel: w469 -> [w475]
                tunnel: w461 -> [w474]
                tunnel: w468 -> [w473]
                tunnel: [w470] -> w467
                tunnel: [w472] -> w466
                tunnel: [w471] -> w465
                stop <- w498 stop-if-true
                n154 = global read "Robot Global Data.vi" "Arm Blue"() -> (w478:dbl)
                n155 = global read "Robot Global Data.vi" "Arm Red"() -> (w489:dbl)
                n156 = Subtract(x=172.089, y=w489) -> (x-y=w476:dbl)
                n157 = Subtract(x=54.2146, y=w478) -> (x-y=w477:dbl)
                n158 = Multiply(x=w477, y=0.5) -> (x*y=w486:dbl)
                n159 = Multiply(x=w476, y=-0.5) -> (x*y=w485:dbl)
                n160 = In Range and Coerce(upper limit=1.0, x=w477, lower limit=-1.0) -> (In Range?=w497:bool)  [unwired: 1 out]
                n161 = In Range and Coerce(upper limit=1.0, x=w476, lower limit=-1.0) -> (In Range?=w496:bool)  [unwired: 1 out]
                n162 = In Range and Coerce(upper limit=0.2, x=w486, lower limit=-0.2) -> (coerced(x)=w481:dbl)  [unwired: 1 out]
                n163 = In Range and Coerce(upper limit=1.0, x=w485, lower limit=-1.0) -> (coerced(x)=w482:dbl)  [unwired: 1 out]
                n164 = call <vilib>:"WPI_MotorControlSetOutput.vi"("Output"=w481, "MotorControlDevRef"=w474) -> ("MotorControlDevRef"=w470:T5)  [unwired: 7 in, 2 out]
                n165 = call <vilib>:"WPI_MotorControlSetOutput.vi"("Output"=w481, "MotorControlDevRef"=w473) -> ("MotorControlDevRef"=w472:T5)  [unwired: 7 in, 2 out]
                n166 = call <vilib>:"WPI_MotorControlSetOutput.vi"("Output"=w482, "MotorControlDevRef"=w475) -> ("MotorControlDevRef"=w471:T5)  [unwired: 7 in, 2 out]
                n167 = And(x=w497, y=w496) -> (x .and. y?=w498:bool)
              }
              n168 = call <vilib>:"WPI_MotorControlSetOutput.vi"("Output"=0.0, "MotorControlDevRef"=w465) -> ()  [unwired: 7 in, 3 out]
              n169 = call <vilib>:"WPI_MotorControlSetOutput.vi"("Output"=0.0, "MotorControlDevRef"=w467) -> ()  [unwired: 7 in, 3 out]
              n170 = call <vilib>:"WPI_MotorControlSetOutput.vi"("Output"=0.0, "MotorControlDevRef"=w466) -> ()  [unwired: 7 in, 3 out]
            }
            frame Enabled {
            }
          }
        }
        frame #2 {
        }
        frame #3 {
          n171 = disable-structure shown="Disabled" {
            disable-tunnel: [w502 _] -> w500
            disable-tunnel: [w501 _] -> w499
            frame Disabled {
              n172 = call <vilib>:"WPI_SolenoidRefNum Registry Get.vi"("refnum name"="Claw") -> ("error out"=w506:errorcluster, "SolenoidDevRef"=w505:T12)  [unwired: 9 in]
              n173 = call-poly <vilib>:"WPI_SolenoidSet.vi"("error in (no error)"=w506, "Value"=WPI_SolenoidValue."On", "SolenoidDevRef"=w505) -> ("error out"=w501:errorcluster, "SolenoidDevRef"=w502:T12)  [unwired: 7 in]
            }
            frame Enabled {
            }
          }
        }
        frame #4 {
          n174 = disable-structure shown="Disabled" {
            frame Disabled {
              n175 = Wait (ms)(milliseconds to wait=u32 500) -> ()  [unwired: 1 out]
            }
            frame Enabled {
            }
          }
        }
        frame #5 {
          n176 = disable-structure shown="Disabled" {
            disable-tunnel: w511 -> [w514 _]
            disable-tunnel: w510 -> [w513 _]
            frame Disabled {
              n177 = call-poly <vilib>:"WPI_SolenoidSet.vi"("error in (no error)"=w513, "Value"=WPI_SolenoidValue."Off", "SolenoidDevRef"=w514) -> ()  [unwired: 7 in, 2 out]
            }
            frame Enabled {
            }
          }
        }
        frame #6 {
          n178 = Tick Count (ms)() -> (millisecond timer value=w517:u32)
        }
        frame #7 {
          n179 = call "Balance.vi"("Start Time"=w520, "Boolean"=TRUE) -> ()  [unwired: 10 in]
        }
        frame #8 {
          n180 = call-poly <vilib>:"WPI_RobotDriveArcadeDrive.vi"("error in (no error)"=w522, "Y axis value"=0.0, "X axis value"=0.0, "RobotDriveDevRef"=w523) -> ()  [unwired: 5 in, 3 out]
        }
      }
    }
    frame "top cube" {
      n181 = flat-sequence {
        tunnel: w555 -> [w576]
        tunnel: w556 -> [w575]
        tunnel: w557 -> [w574]
        tunnel: [w576] -> w544
        tunnel: [w564] -> w538
        tunnel: [w575] -> w537
        tunnel: [w574] -> w536
        tunnel: w535 -> [w561]
        tunnel: w534 -> [w571]
        tunnel: w533 -> [w568]
        tunnel: w532 -> [w565]
        tunnel: [w563] -> w526
        tunnel: w544 -> [w581]
        tunnel: [w580] -> w539
        tunnel: w538 -> [w580]
        tunnel: w537 -> [w578]
        tunnel: w536 -> [w579]
        tunnel: [w577] -> w527
        tunnel: w526 -> [w577]
        tunnel: [w621] -> w540
        tunnel: w539 -> [w621]
        tunnel: [w620] -> w528
        tunnel: w527 -> [w620]
        tunnel: [w625] -> w554
        tunnel: [w624] -> w552
        tunnel: [w623] -> w541
        tunnel: w540 -> [w623]
        tunnel: [w622] -> w529
        tunnel: w528 -> [w622]
        tunnel: w554 -> [w635]
        tunnel: [w635] -> w553
        tunnel: w552 -> [w634]
        tunnel: [w634] -> w551
        tunnel: [w633] -> w542
        tunnel: w541 -> [w633]
        tunnel: [w632] -> w530
        tunnel: w529 -> [w632]
        tunnel: w553 -> [w640]
        tunnel: w551 -> [w639]
        tunnel: [w638] -> w543
        tunnel: w542 -> [w638]
        tunnel: [w637] -> w531
        tunnel: w530 -> [w637]
        tunnel: [w649] -> w548
        tunnel: [w648] -> w547
        tunnel: w550 -> [w647]
        tunnel: w549 -> [w646]
        tunnel: w543 -> [w645]
        tunnel: w531 -> [w644]
        tunnel: w548 -> [w665]
        tunnel: w547 -> [w664]
        tunnel: [w663] -> w546
        tunnel: [w662] -> w545
        tunnel: w546 -> [w678]
        tunnel: w545 -> [w677]
        frame #0 {
          n182 = Wait (ms)(milliseconds to wait=u32 30) -> ()  [unwired: 1 out]
          n183 = call <vilib>:"Spark MAX Set Sensor Position.vi"("Sensor Type (Hall Sensor)"=Spark_MAX_Sensor_Type."Hall Sensor", "Position"=0.0, "MotorControlDeviceRef"=w561) -> ("MotorControlDeviceRef"=w560:T5)  [unwired: 7 in, 1 out]
          n184 = call <vilib>:"Spark MAX Set Sensor Position.vi"("Sensor Type (Hall Sensor)"=Spark_MAX_Sensor_Type."Hall Sensor", "Position"=0.0, "MotorControlDeviceRef"=w565) -> ()  [unwired: 7 in, 2 out]
          n185 = call <vilib>:"Spark MAX Get Sensor Position.vi"("MotorControlDevRef in"=w560) -> ("Sensor Position"=w563:dbl, "MotorControlDevRef out"=w564:T5)  [unwired: 7 in, 2 out]
          n186 = call <vilib>:"Spark MAX Set Sensor Position.vi"("Sensor Type (Hall Sensor)"=Spark_MAX_Sensor_Type."Hall Sensor", "Position"=0.0, "MotorControlDeviceRef"=w568) -> ()  [unwired: 7 in, 2 out]
          n187 = call <vilib>:"Spark MAX Set Sensor Position.vi"("Sensor Type (Hall Sensor)"=Spark_MAX_Sensor_Type."Hall Sensor", "Position"=0.0, "MotorControlDeviceRef"=w571) -> ()  [unwired: 7 in, 2 out]
        }
        frame #1 {
          n188 = disable-structure shown="Disabled" {
            disable-tunnel: w579 -> [w590 _]
            disable-tunnel: [w582 _] -> _
            disable-tunnel: w581 -> [w589 _]
            disable-tunnel: w578 -> [w582 _]
            frame Disabled {
              n189 = while {
                tunnel: w590 -> [w596]
                tunnel: w582 -> [w595]
                tunnel: w589 -> [w594]
                tunnel: [w591] -> w588
                tunnel: [w593] -> w587
                tunnel: [w592] -> w586
                stop <- w619 stop-if-true
                n190 = global read "Robot Global Data.vi" "Arm Blue"() -> (w599:dbl)
                n191 = global read "Robot Global Data.vi" "Arm Red"() -> (w610:dbl)
                n192 = Subtract(x=172.089, y=w610) -> (x-y=w597:dbl)
                n193 = Subtract(x=54.2146, y=w599) -> (x-y=w598:dbl)
                n194 = Multiply(x=w598, y=0.5) -> (x*y=w607:dbl)
                n195 = Multiply(x=w597, y=-0.5) -> (x*y=w606:dbl)
                n196 = In Range and Coerce(upper limit=1.0, x=w598, lower limit=-1.0) -> (In Range?=w618:bool)  [unwired: 1 out]
                n197 = In Range and Coerce(upper limit=1.0, x=w597, lower limit=-1.0) -> (In Range?=w617:bool)  [unwired: 1 out]
                n198 = In Range and Coerce(upper limit=0.2, x=w607, lower limit=-0.2) -> (coerced(x)=w602:dbl)  [unwired: 1 out]
                n199 = In Range and Coerce(upper limit=1.0, x=w606, lower limit=-1.0) -> (coerced(x)=w603:dbl)  [unwired: 1 out]
                n200 = call <vilib>:"WPI_MotorControlSetOutput.vi"("Output"=w602, "MotorControlDevRef"=w595) -> ("MotorControlDevRef"=w591:T5)  [unwired: 7 in, 2 out]
                n201 = call <vilib>:"WPI_MotorControlSetOutput.vi"("Output"=w602, "MotorControlDevRef"=w594) -> ("MotorControlDevRef"=w593:T5)  [unwired: 7 in, 2 out]
                n202 = call <vilib>:"WPI_MotorControlSetOutput.vi"("Output"=w603, "MotorControlDevRef"=w596) -> ("MotorControlDevRef"=w592:T5)  [unwired: 7 in, 2 out]
                n203 = And(x=w618, y=w617) -> (x .and. y?=w619:bool)
              }
              n204 = call <vilib>:"WPI_MotorControlSetOutput.vi"("Output"=0.0, "MotorControlDevRef"=w586) -> ()  [unwired: 7 in, 3 out]
              n205 = call <vilib>:"WPI_MotorControlSetOutput.vi"("Output"=0.0, "MotorControlDevRef"=w588) -> ()  [unwired: 7 in, 3 out]
              n206 = call <vilib>:"WPI_MotorControlSetOutput.vi"("Output"=0.0, "MotorControlDevRef"=w587) -> ()  [unwired: 7 in, 3 out]
            }
            frame Enabled {
            }
          }
        }
        frame #2 {
        }
        frame #3 {
          n207 = disable-structure shown="Disabled" {
            disable-tunnel: [w627 _] -> w625
            disable-tunnel: [w626 _] -> w624
            frame Disabled {
              n208 = call <vilib>:"WPI_SolenoidRefNum Registry Get.vi"("refnum name"="Claw") -> ("error out"=w631:errorcluster, "SolenoidDevRef"=w630:T12)  [unwired: 9 in]
              n209 = call-poly <vilib>:"WPI_SolenoidSet.vi"("error in (no error)"=w631, "Value"=WPI_SolenoidValue."On", "SolenoidDevRef"=w630) -> ("error out"=w626:errorcluster, "SolenoidDevRef"=w627:T12)  [unwired: 7 in]
            }
            frame Enabled {
            }
          }
        }
        frame #4 {
          n210 = disable-structure shown="Disabled" {
            frame Disabled {
              n211 = Wait (ms)(milliseconds to wait=u32 500) -> ()  [unwired: 1 out]
            }
            frame Enabled {
            }
          }
        }
        frame #5 {
          n212 = disable-structure shown="Disabled" {
            disable-tunnel: w640 -> [w643 _]
            disable-tunnel: w639 -> [w642 _]
            frame Disabled {
              n213 = call-poly <vilib>:"WPI_SolenoidSet.vi"("error in (no error)"=w642, "Value"=WPI_SolenoidValue."Off", "SolenoidDevRef"=w643) -> ()  [unwired: 7 in, 2 out]
            }
            frame Enabled {
            }
          }
        }
        frame #6 {
          # "+ x is backward in autonomous"
          n214 = while {
            tunnel: [w659] -> w649
            tunnel: [w658] -> w648
            tunnel: w647 -> [w656]
            tunnel: w646 -> [w655]
            tunnel: w645 -> [w653]
            tunnel: w644 -> [w650]
            tunnel: [w650] -> _
            stop <- w657 stop-if-true
            # "198"
            # "makes it drive straight back"
            n215 = call <vilib>:"Spark MAX Get Sensor Position.vi"("MotorControlDevRef in"=w653) -> ("Sensor Position"=w651:dbl)  [unwired: 7 in, 3 out]
            "Sensor Position 3" <- w651
            n216 = call-poly <vilib>:"WPI_RobotDriveArcadeDrive.vi"("error in (no error)"=w655, "Y axis value"=0.0, "X axis value"=0.7, "RobotDriveDevRef"=w656) -> ("error out"=w658:errorcluster, "RobotDriveDevRef"=w659:T4)  [unwired: 5 in, 1 out]
            n217 = Subtract(x=w651, y=w650) -> (x-y=w652:dbl)
            "Right Drive Encoder 3" <- w652
            n218 = Greater?(x=w652, y=198.0) -> (0:w657:bool)
          }
          "Timestamp 3" <- w644
        }
        frame #7 {
          n219 = while {
            tunnel: w665 -> [w674]
            tunnel: w664 -> [w673]
            tunnel: [w672] -> w663
            tunnel: [w671] -> w662
            stop <- w666 stop-if-true
            n220 = global read "Robot Global Data.vi" "Real Yaw"() -> (w668:dbl)
            "Real Yaw 2" <- w668
            n221 = call-poly <vilib>:"WPI_RobotDriveArcadeDrive.vi"("error in (no error)"=w673, "Y axis value"=0.4, "X axis value"=0.0, "RobotDriveDevRef"=w674) -> ("error out"=w671:errorcluster, "RobotDriveDevRef"=w672:T4)  [unwired: 5 in, 1 out]
            n222 = In Range and Coerce(upper limit=170.0, x=w668, lower limit=-170.0) -> (In Range?=w667:bool)  [unwired: 1 out]
            n223 = Not(x=w667) -> (.not. x?=w666:bool)
          }
        }
        frame #8 {
          n224 = call-poly <vilib>:"WPI_RobotDriveArcadeDrive.vi"("error in (no error)"=w677, "Y axis value"=0.0, "X axis value"=0.0, "RobotDriveDevRef"=w678) -> ()  [unwired: 5 in, 3 out]
        }
      }
    }
    frame "Balance" {
      # "You can put your main auto here, or you can right-click on the case and make any\nother frame be the default case."
      # "This is the frame that will execute if no selection is made, or if it is not recognized"
      n225 = flat-sequence {
        tunnel: [w682] -> w681
        tunnel: w681 -> [w684]
        frame #0 {
          n226 = Tick Count (ms)() -> (millisecond timer value=w682:u32)
        }
        frame #1 {
          n227 = call "Balance.vi"("Start Time"=w684, "Boolean"=TRUE) -> ()  [unwired: 10 in]
        }
      }
    }
    frame "Drive Straight" {
      n228 = flat-sequence {
        tunnel: [w690] -> w687
        tunnel: w686 -> [w690]
        tunnel: [w696] -> w689
        tunnel: [w695] -> w688
        tunnel: w687 -> [w693]
        tunnel: w685 -> [w692]
        tunnel: w689 -> [w709]
        tunnel: w688 -> [w708]
        frame #0 {
          # "Creates the starting angle"
          n229 = global read "Robot Global Data.vi" "yaw"() -> (w691:dbl)
          n230 = global write "Robot Global Data.vi" "Gyro Starting Value in our match"(w691) -> ()
        }
        frame #1 {
          n231 = Tick Count (ms)() -> (millisecond timer value=w694:u32)
          n232 = while {
            tunnel: [w706] -> w696
            tunnel: [w705] -> w695
            tunnel: w694 -> [w703]
            tunnel: w693 -> [w698]
            tunnel: w692 -> [w697]
            stop <- w699 stop-if-true
            n233 = call "Drive straight.vi"("Start Time"=w703, "Length(seconds)"=6.0, "Desired angle"=0.0) -> ("Complete or not"=w699:bool, "X Power"=w700:dbl)  [unwired: 7 in]
            n234 = Wait (ms)(milliseconds to wait=u32 10) -> ()  [unwired: 1 out]
            n235 = call-poly <vilib>:"WPI_RobotDriveArcadeDrive.vi"("error in (no error)"=w697, "Y axis value"=-0.55, "X axis value"=w700, "RobotDriveDevRef"=w698) -> ("error out"=w705:errorcluster, "RobotDriveDevRef"=w706:T4)  [unwired: 5 in, 1 out]
          }
        }
        frame #2 {
          n236 = call-poly <vilib>:"WPI_RobotDriveArcadeDrive.vi"("error in (no error)"=w708, "Y axis value"=0.0, "X axis value"=0.0, "RobotDriveDevRef"=w709) -> ()  [unwired: 5 in, 3 out]
        }
      }
    }
    frame "Test Balance" {
      n237 = flat-sequence {
        tunnel: w715 -> [w719]
        tunnel: w714 -> [w718]
        tunnel: [w717] -> w713
        tunnel: [w716] -> w712
        tunnel: w713 -> [w732]
        tunnel: w712 -> [w731]
        frame #0 {
          n238 = while {
            shift-right: [w725] -> w716
            shift-left: w719 -> [w728]
            shift-right: [w726] -> w717
            shift-left: w718 -> [w727]
            stop <- w720 stop-if-true
            n239 = global read "Robot Global Data.vi" "Pitch"() -> (w722:dbl)
            n240 = call-poly <vilib>:"WPI_RobotDriveArcadeDrive.vi"("error in (no error)"=w727, "Y axis value"=-0.55, "X axis value"=0.0, "RobotDriveDevRef"=w728) -> ("error out"=w726:errorcluster, "RobotDriveDevRef"=w725:T4)  [unwired: 5 in, 1 out]
            n241 = In Range and Coerce(upper limit=10.0, x=w722, lower limit=-10.0 ("y")) -> (In Range?=w723:bool)  [unwired: 1 out]
            n242 = Not(x=w723) -> (.not. x?=w720:bool)
          }
        }
        frame #1 {
          n243 = while {
            tunnel: w732 -> [w734]
            tunnel: w731 -> [w733]
            stop <- FALSE stop-if-true
            n244 = call "Derivative balance.vi"() -> ("Motor Power"=w737:dbl)  [unwired: 11 in]
            n245 = call-poly <vilib>:"WPI_RobotDriveArcadeDrive.vi"("error in (no error)"=w734, "Y axis value"=w737, "X axis value"=0.0, "RobotDriveDevRef"=w733) -> ()  [unwired: 5 in, 3 out]
          }
        }
      }
    }
    frame Default {
    }
  }
